vi "Write Then Read.vi"(8 "error in (no error)":errorcluster, 10 "Parameter 1":string="VE", 11 "LifterTCP in":refnum<class "LifterTCP.lvclass">) -> (0 "error out":errorcluster, 2 "Read Data":string, 3 "LifterTCP out":refnum<class "LifterTCP.lvclass">)   [LabVIEW 2019, in "LifterTCP.lvclass"]
uses:
  LifterTCP.lvclass
  LifterTCP.lvclass/LifterTCP.ctl
panel:
  out "Data error count":dbl
  out "TCP Error count":dbl
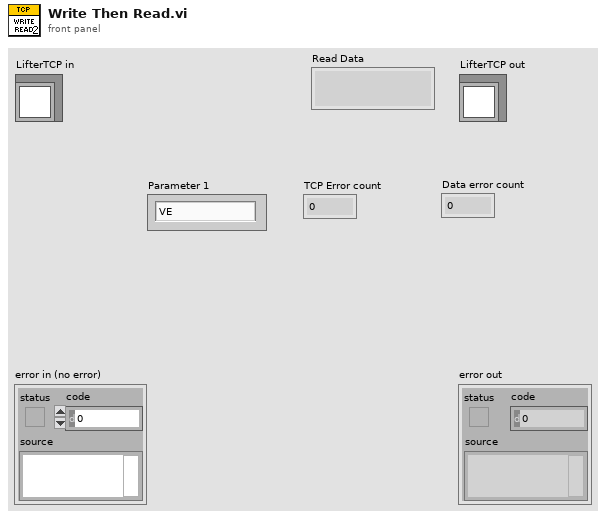
[diagram p1: front panel]
types:
  T1 = typedef "Semaphore RefNum" = refnum<k1>
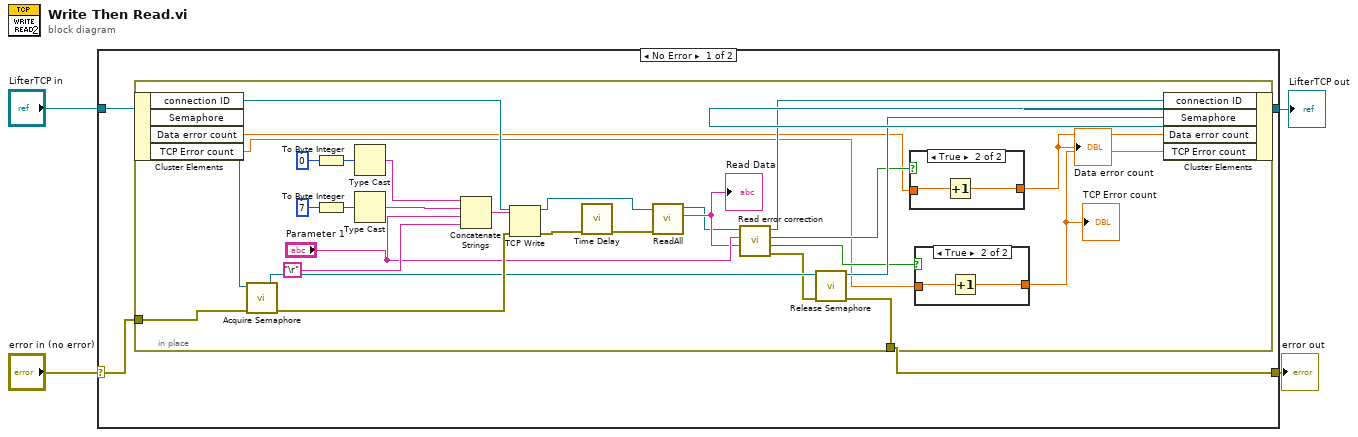
[diagram p0: block diagram]
diagram:
  n1 = case shown="No Error" "error in (no error)" {
    selector: "error in (no error)" -> [w6 w45]
    tunnel: [w5 w45] -> w3
    tunnel: [w7 w44] -> w1
    tunnel: "LifterTCP in" -> [w8 w44]
    frame No Error {
      n2 = in-place {
        in-place-border: w6 -> [w27]
        in-place-border: [w15] -> w5
        n3 = in-place-cluster #1(w8) -> ("connection ID"=w21:refnum<k5>, "Semaphore"=w28:T1, "Data error count"=w13:dbl, "TCP Error count"=w10:dbl)
        n4 = call <vilib>:"Acquire Semaphore.vi"("error in (no error)"=w27, "semaphore"=w28) -> ("error out"=w26:errorcluster, "semaphore out"=w22:T1)  [unwired: 3 in, 1 out]
        n5 = To Byte Integer(number=i8 0) -> (8bit integer=w34:i8)
        n6 = To Byte Integer(number=i8 7) -> (8bit integer=w37:i8)
        n7 = Type Cast(x=w34) -> (*(type *) &x=w35:string)  [unwired: 1 in]
        n8 = Type Cast(x=w37) -> (*(type *) &x=w36:string)  [unwired: 1 in]
        n9 = Concatenate Strings(w35, w36, "Parameter 1", "\r") -> (w29:string)
        n10 = TCP Write(connection ID=w21, data in=w29, error in (no error)=w26) -> (connection ID out=w23:refnum<k5>, error out=w30:errorcluster)  [unwired: 1 in, 1 out]
        n11 = call "Time Delay"("error in (no error)"=w30) -> ("error out"=w24:errorcluster)  [unwired: 10 in]
        n12 = call "ReadAll.vi"("error in (no error)"=w24, "connection ID"=w23) -> ("Read Data"=w19:string, "connection ID out"=w18:refnum<k5>)  [unwired: 7 in, 1 out]
        "Read Data" <- w19
        n13 = call "Read error correction.vi"("Recieve data"=w19, "Sent command header"="Parameter 1", "connection ID"=w18) -> ("error out"=w16:errorcluster, "TCP Error"=w11:bool, "Data Error"=w14:bool, "connection ID out"=w17:refnum<k5>)  [unwired: 5 in]
        n14 = call <vilib>:"Release Semaphore.vi"("error in (no error)"=w16, "semaphore"=w22) -> ("error out"=w15:errorcluster, "semaphore out"=w25:T1)  [unwired: 4 in]
        n15 = case shown="True" w14 {
          tunnel: w13 -> [w41 w43]
          tunnel: [w41 w42] -> w12
          frame False {
          }
          frame True {
            n16 = Increment(x=w43) -> (x+1=w42:dbl)
          }
        }
        "Data error count" <- w12
        n17 = case shown="True" w11 {
          tunnel: w10 -> [w38 w40]
          tunnel: [w38 w39] -> w9
          frame False {
          }
          frame True {
            n18 = Increment(x=w40) -> (x+1=w39:dbl)
          }
        }
        "TCP Error count" <- w9
        n19 = in-place-cluster #1("connection ID"=w17, "Semaphore"=w25, "Data error count"=w12, "TCP Error count"=w9) -> (w7:refnum<class "LifterTCP.lvclass">)
      }
    }
    frame Error {
    }
  }
  "error out" <- w3
  "LifterTCP out" <- w1
